vi "Func1.vi"(8 "error in (no error)":errorcluster, 11 "Subject in":refnum<class "Subject.lvclass">) -> (0 "error out":errorcluster, 3 "Subject out":refnum<class "Subject.lvclass">)   [LabVIEW 2014, in "forcible Proxy.lvlib" / "Subject.lvclass"]
uses:
  Subject.lvclass
  Subject.lvclass/Subject.ctl
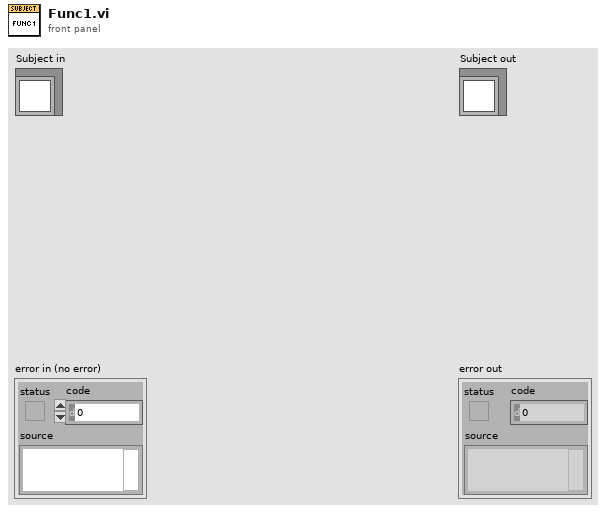
[diagram p1: front panel]
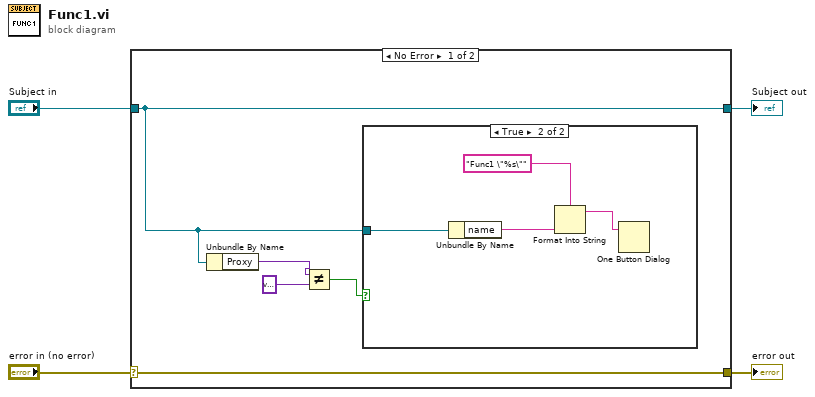
[diagram p0: block diagram]
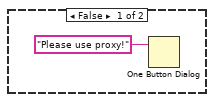
[diagram p2: hidden frame]
diagram:
  n1 = case shown="No Error" "error in (no error)" {
    selector: "error in (no error)" -> [w9 w16]
    tunnel: [w9 w16] -> w3
    tunnel: [w8 w15] -> w1
    tunnel: "Subject in" -> [w8 w15]
    frame No Error {
      n2 = Unbundle By Name(w8) -> ("Proxy"=w7:variant)
      n3 = Not Equal?(x=w7, y=variant) -> (x != y?=w5:bool)
      n4 = case shown="True" w5 {
        tunnel: w8 -> [_ w11]
        frame False {
          n5 = One Button Dialog(message="Please use proxy!") -> ()  [unwired: 1 in, 1 out]
        }
        frame True {
          n6 = Unbundle By Name(w11) -> ("name"=w14:string)
          n7 = Format Into String(format string="Func1 \"%s\"", w14) -> (resulting string=w12:string)  [unwired: 2 in, 1 out]
          n8 = One Button Dialog(message=w12) -> ()  [unwired: 1 in, 1 out]
        }
      }
    }
    frame Error {
    }
  }
  "error out" <- w3
  "Subject out" <- w1
